vi "SwissSPAD Live_Init Settings.vi"(8 "error in (no error)":errorcluster) -> (0 "error out":errorcluster)   [LabVIEW 2021]
uses:
  SwissSPAD Live_Settings List.ctl
  SwissSPAD Live_SS2 Gate Configuration.ctl
  SwissSPAD Live_SS2 Gate Definition.ctl
  SwissSPAD Live_Gate Configuration Action.ctl
  SwissSPAD Live_SS2 DAQ Parameters 3.ctl
  SwissSPAD Live_SS3 DAQ Parameters.ctl
  SwissSPAD Live_SS3 Gate Definition.ctl
  SS3 Gate Width Definition Mode.ctl
  SwissSPAD Live_File Information.ctl
  SwissSPAD Live_FPGA Data to Display.ctl
  Phasor/Image Binning Options.ctl
  SwissSPAD Live_Image Display Options.ctl
  SwissSPAD Live_Image ROI Information.ctl
  SwissSPAD Live_SS3 Displayed Image.ctl
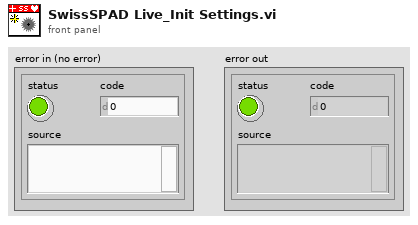
[diagram p1: front panel]
types:
  T1 = typedef "SwissSPAD Live_SS2 Gate Configuration.ctl" = cluster{"Gate Configuration":string, "Gate Offset":u32, "Gate Definition":T2}
  T2 = typedef "SwissSPAD Live_SS2 Gate Definition.ctl" = cluster{"gs_psincdec_0":u32, "gs_psincdec_1":u32, "gs_psincdec_2":u32, "gs_psincdec_3":u32, "gs_no_shift_adj_1":u32, "gs_no_shift_adj_2":u32, "gs_no_shift_adj_3":u32}
  T3 = typedef "SwissSPAD Live_Settings List.ctl" = enum16{"FPGA:Bottom Half", "FPGA:Top Half", "FPGA:Bottom Bitfile Path", "FPGA:Top Bitfile Path", "FPGA:Bottom Bitstream Version", "FPGA:Top Bitstream Version", "FPGA:Auto Reset FPGA", "FPGA:Bottom FPGA Serial Number", "FPGA:Top FPGA Serial Number", "FPGA:Detector PCB Version", "Acquisition Parameters:Microlens", "Acquisition Parameters:SS2 DAQ Parameters", "Acquisition Parameters:Gate Configuration Array", "Acquisition Parameters:SS3 DAQ Parameters", "Acquisition Parameters:Buffer Size (# 8-bit Gates)", "File Information:File Information", "File Information:# Datasets in Series", "File Information:Scrambled File Flag", "File Information:SS3 Gate Slip Correction", "File Information:SS3 Hot Pixel Mismatch Detection", "File Information:Delay between Datasets", "File Information:Save Sum of All Gates Preview", "Image Parameters:Image ROI Information", "Image Parameters:Image Binning Options", "Image Parameters:SS3 Displayed Image", "Image Parameters:Image Display Options", "Image Parameters:Use Histogram Cursors", "Image Parameter:FPGA Data to Display", "UI Settings:Histogram Bins Number", "UI Settings:Use Image Display Options", "UI Settings:Verbose Settings", "UI Settings:Verbose Saving"}
  T4 = typedef "SwissSPAD Live_Gate Configuration Action.ctl" = enum16{"Get Gate Configuration Name", "Get Configuration by Name", "Add Gate Configuration", "Delete Gate Configuration", "Rename Gate Configuration"}
  T5 = typedef "SwissSPAD Live_SS2 DAQ Parameters 3.ctl" = cluster{"10 bits":bool, "# Exposure Sequences":u32, "# 1-bit Frame per Gate":u32, "Gate Shift":u32, "# Gates per Set":u32, "# Sets":u32, "Laser Period":dbl[unit], "Sync Period":dbl[unit], "Gate Offset":u32, "Auto-adjust Gate Offset":bool, "Gate Definition":T2, "Reversed Shift":bool}
  T6 = typedef "SwissSPAD Live_SS3 DAQ Parameters.ctl" = cluster{"10 bits":bool, "# Exposure Sequences":u32, "# 1-bit Frame per Gate":u32, "Gate Shift":u32, "# Gate Pairs per Set":u32, "# Sets":u32, "Laser Period":dbl[unit], "Sync Period":dbl[unit], "Gate Offset":u32, "Auto-adjust Gate Offset":bool, "Gate Definition":T7, "Gate Width (ns)":dbl, "Reversed Shift":bool, "Intensity Mode":bool, "Gate Definition Mode":T8}
  T7 = typedef "SwissSPAD Live_SS3 Gate Definition.ctl" = cluster{"gs_psincdec_0":u32, "gs_psincdec_1":u32, "gs_no_shift_adj_1":u32, "gate_adj_2":u32}
  T8 = typedef "SS3 Gate Width Definition Mode.ctl" = enum32{"Item 0", "Item 1"}
  T9 = typedef "SwissSPAD Live_File Information.ctl" = cluster{"File Folder":path, "File Name":string, "File Index":u32, "Author":string, "Sample":string, "Compression":bool, "Compression Level":u8}
  T10 = typedef "SwissSPAD Live_FPGA Data to Display.ctl" = enum16{"Bottom FPGA", "Top FPGA", "Both"}
  T11 = typedef "Image Binning Options.ctl" = cluster{"Use Image Binning":bool, "X Bin":i32, "Y Bin":i32}
  T12 = typedef "SwissSPAD Live_Image Display Options.ctl" = cluster{"Remove Screamers":bool, "Delta":sgl, "Equalize Histogram":bool, "Percentile":sgl, "Hot Pixel Mask Image":path, "Use Hot Pixel Mask":bool}
  T13 = typedef "SwissSPAD Live_Image ROI Information.ctl" = cluster{"Save ROI Only":bool, "Left":u16, "Top":u16, "Right":u16, "Bottom":u16, "Use Current ROI":bool}
  T14 = typedef "SwissSPAD Live_SS3 Displayed Image.ctl" = enum16{"Gate 1", "Gate 2", "Gate 1 + Gate 2"}
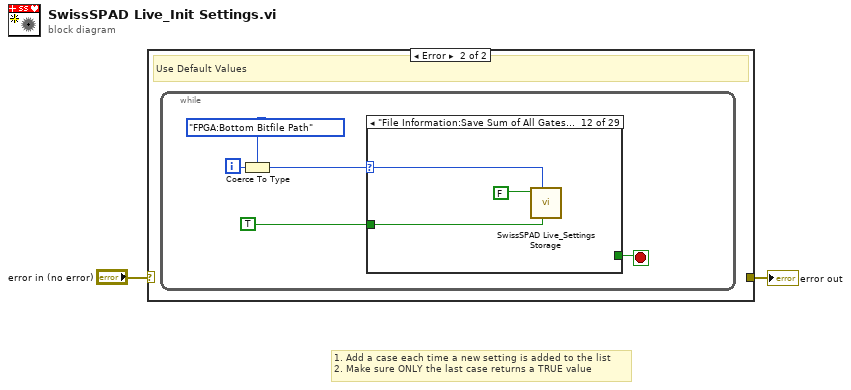
[diagram p0: block diagram]
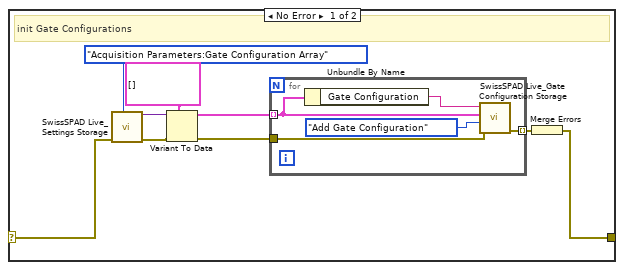
[diagram p2: hidden frame]
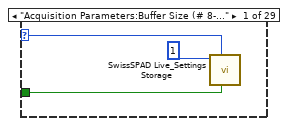
[diagram p3: hidden frame]
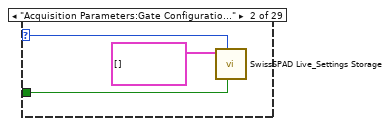
[diagram p4: hidden frame]
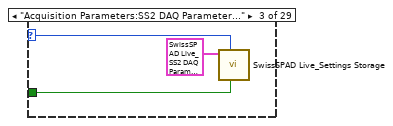
[diagram p5: hidden frame]
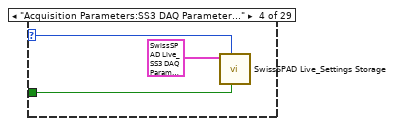
[diagram p6: hidden frame]
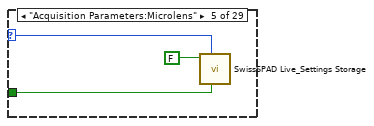
[diagram p7: hidden frame]
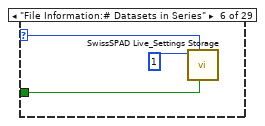
[diagram p8: hidden frame]
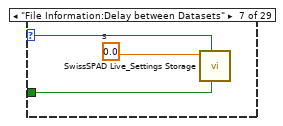
[diagram p9: hidden frame]
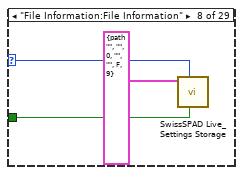
[diagram p10: hidden frame]
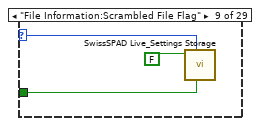
[diagram p11: hidden frame]
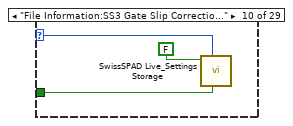
[diagram p12: hidden frame]
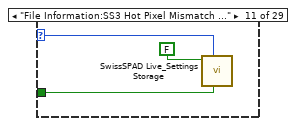
[diagram p13: hidden frame]
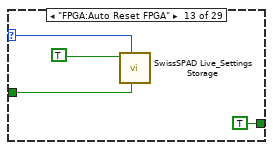
[diagram p14: hidden frame]
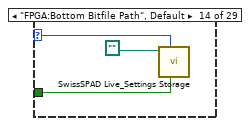
[diagram p15: hidden frame]
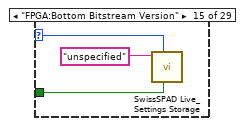
[diagram p16: hidden frame]
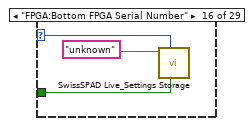
[diagram p17: hidden frame]
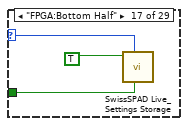
[diagram p18: hidden frame]
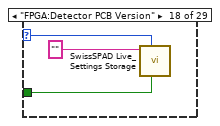
[diagram p19: hidden frame]
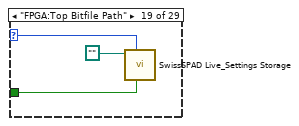
[diagram p20: hidden frame]
diagram:
  # "1. Add a case each time a new setting is added to the list\n2. Make sure ONLY the last case returns a TRUE value"
  n1 = case shown="Error" "error in (no error)" {
    selector: "error in (no error)" -> [w6 _]
    tunnel: [w5 _] -> w1
    frame No Error {
      # "init Gate Configurations"
      n2 = call "SwissSPAD Live_Settings Storage.vi"("Settings List"=SwissSPAD_Live_Settings_List."Acquisition Parameters:Gate Configuration Array", "Error In"=w6) -> ("Error Out"=w11:errorcluster, "Variant Data out"=w3:variant)  [unwired: 8 in]
      n3 = Variant To Data(error in=w11, type=T1[] [] ("Gate Configuration Definitions"), Variant=w3) -> (data=w9:T1[], error out=w8:errorcluster)
      n4 = for {
        tunnel: w9 -> [w15] mode=indexing
        tunnel: w8 -> [w13]
        tunnel: [w12] -> w7 mode=indexing
        n5 = Unbundle By Name(w15) -> ("Gate Configuration"=w16:string)
        n6 = call "SwissSPAD Live_Gate Configuration Storage.vi"("Error In"=w13, "Action"=SwissSPAD_Live_Gate_Configuration_Action."Add Gate Configuration", "Gate Configuration Definition in"=w15, "Gate Configuration Name in"=w16) -> ("Error Out"=w12:errorcluster)  [unwired: 2 in, 5 out]
      }
      n7 = Merge Errors(w7) -> (w5:errorcluster)
    }
    frame Error {
      # "Use Default Values"
      n8 = while {
        i -> [w21]
        stop <- w17 stop-if-true
        n9 = Coerce To Type(0:w21, 1:SwissSPAD_Live_Settings_List."FPGA:Bottom Bitfile Path" ("Settings List")) -> (2:w19:T3)
        n10 = case shown="\"File Information:Save Sum of All Gates Preview\"" w19 {
          selector: w19 -> [w23 w25 w29 w31 w35 w38 w41 w43 w47 w50 w53 w56 w58 w63 w66 w69 w72 w74 w78 w81 w84 w87 w90 w93 w95 w99 w102 w105 w108]
          tunnel: TRUE -> [w24 w27 w30 w33 w36 w39 w42 w45 w48 w51 w54 w57 w60 w64 w67 w70 w73 w76 w79 w82 w85 w88 w91 w94 w97 w100 w103 w106 w109]
          tunnel: [_ _ _ _ _ _ _ _ _ _ _ _ TRUE _ _ _ _ _ _ _ _ _ _ _ _ _ _ _ _] -> w17
          frame "Acquisition Parameters:Buffer Size (# 8-bit Gates)" {
            n11 = call "SwissSPAD Live_Settings Storage.vi"("Set/Get(F)"=w24, "Settings List"=w23, "Variant Data in"=u32 1 ("Buffer Size #Gates)")) -> ()  [unwired: 7 in, 2 out]
          }
          frame "Acquisition Parameters:Gate Configuration Array" {
            n12 = call "SwissSPAD Live_Settings Storage.vi"("Set/Get(F)"=w27, "Settings List"=w25, "Variant Data in"=T1[] [] ("Gate Configuration Definitions")) -> ()  [unwired: 7 in, 2 out]
          }
          frame "Acquisition Parameters:SS2 DAQ Parameters" {
            n13 = call "SwissSPAD Live_Settings Storage.vi"("Set/Get(F)"=w30, "Settings List"=w29, "Variant Data in"=T5 {"10 bits"=FALSE, "# Exposure Sequences"=100, "# 1-bit Frame per Gate"=255, "Gate Shift"=0, "# Gates per Set"=1, "# Sets"=1, "Laser Period"=0.0, "Sync Period"=0.0, "Gate Offset"=650, "Auto-adjust Gate Offset"=FALSE, "Gate Definition"={"gs_psincdec_0"=1, "gs_psincdec_1"=0, "gs_psincdec_2"=0, "gs_psincdec_3"=0, "gs_no_shift_adj_1"=65, "gs_no_shift_adj_2"=90, "gs_no_shift_adj_3"=30}, "Reversed Shift"=FALSE} ("SS2 DAQ Parameters")) -> ()  [unwired: 7 in, 2 out]
          }
          frame "Acquisition Parameters:SS3 DAQ Parameters" {
            n14 = call "SwissSPAD Live_Settings Storage.vi"("Set/Get(F)"=w33, "Settings List"=w31, "Variant Data in"=T6 {"10 bits"=FALSE, "# Exposure Sequences"=0, "# 1-bit Frame per Gate"=255, "Gate Shift"=0, "# Gate Pairs per Set"=0, "# Sets"=1, "Laser Period"=0.0, "Sync Period"=0.0, "Gate Offset"=0, "Auto-adjust Gate Offset"=FALSE, "Gate Definition"={"gs_psincdec_0"=0, "gs_psincdec_1"=0, "gs_no_shift_adj_1"=0, "gate_adj_2"=0}, "Gate Width (ns)"=0.0, "Reversed Shift"=FALSE, "Intensity Mode"=FALSE, "Gate Definition Mode"=enum."Item 0"} ("SS3 DAQ Parameters")) -> ()  [unwired: 7 in, 2 out]
          }
          frame "Acquisition Parameters:Microlens" {
            n15 = call "SwissSPAD Live_Settings Storage.vi"("Set/Get(F)"=w36, "Settings List"=w35, "Variant Data in"=FALSE) -> ()  [unwired: 7 in, 2 out]
          }
          frame "File Information:# Datasets in Series" {
            n16 = call "SwissSPAD Live_Settings Storage.vi"("Set/Get(F)"=w39, "Settings List"=w38, "Variant Data in"=1) -> ()  [unwired: 7 in, 2 out]
          }
          frame "File Information:Delay between Datasets" {
            w40 = dbl[unit] 0.0  # s
            n17 = call "SwissSPAD Live_Settings Storage.vi"("Set/Get(F)"=w42, "Settings List"=w41, "Variant Data in"=w40) -> ()  [unwired: 7 in, 2 out]
          }
          frame "File Information:File Information" {
            n18 = call "SwissSPAD Live_Settings Storage.vi"("Set/Get(F)"=w45, "Settings List"=w43, "Variant Data in"=T9 {"File Folder"=path "", "File Name"="", "File Index"=0, "Author"="", "Sample"="", "Compression"=FALSE, "Compression Level"=9} ("File Information")) -> ()  [unwired: 7 in, 2 out]
          }
          frame "File Information:Scrambled File Flag" {
            n19 = call "SwissSPAD Live_Settings Storage.vi"("Set/Get(F)"=w48, "Settings List"=w47, "Variant Data in"=FALSE) -> ()  [unwired: 7 in, 2 out]
          }
          frame "File Information:SS3 Gate Slip Correction" {
            n20 = call "SwissSPAD Live_Settings Storage.vi"("Set/Get(F)"=w51, "Settings List"=w50, "Variant Data in"=FALSE) -> ()  [unwired: 7 in, 2 out]
          }
          frame "File Information:SS3 Hot Pixel Mismatch Detection" {
            n21 = call "SwissSPAD Live_Settings Storage.vi"("Set/Get(F)"=w54, "Settings List"=w53, "Variant Data in"=FALSE) -> ()  [unwired: 7 in, 2 out]
          }
          frame "File Information:Save Sum of All Gates Preview" {
            n22 = call "SwissSPAD Live_Settings Storage.vi"("Set/Get(F)"=w57, "Settings List"=w56, "Variant Data in"=FALSE) -> ()  [unwired: 7 in, 2 out]
          }
          frame "FPGA:Auto Reset FPGA" {
            n23 = call "SwissSPAD Live_Settings Storage.vi"("Set/Get(F)"=w60, "Settings List"=w58, "Variant Data in"=TRUE) -> ()  [unwired: 7 in, 2 out]
          }
          frame "FPGA:Bottom Bitfile Path", Default {
            n24 = call "SwissSPAD Live_Settings Storage.vi"("Set/Get(F)"=w64, "Settings List"=w63, "Variant Data in"=path "") -> ()  [unwired: 7 in, 2 out]
          }
          frame "FPGA:Bottom Bitstream Version" {
            n25 = call "SwissSPAD Live_Settings Storage.vi"("Set/Get(F)"=w67, "Settings List"=w66, "Variant Data in"="unspecified") -> ()  [unwired: 7 in, 2 out]
          }
          frame "FPGA:Bottom FPGA Serial Number" {
            n26 = call "SwissSPAD Live_Settings Storage.vi"("Set/Get(F)"=w70, "Settings List"=w69, "Variant Data in"="unknown") -> ()  [unwired: 7 in, 2 out]
          }
          frame "FPGA:Bottom Half" {
            n27 = call "SwissSPAD Live_Settings Storage.vi"("Set/Get(F)"=w73, "Settings List"=w72, "Variant Data in"=TRUE) -> ()  [unwired: 7 in, 2 out]
          }
          frame "FPGA:Detector PCB Version" {
            n28 = call "SwissSPAD Live_Settings Storage.vi"("Set/Get(F)"=w76, "Settings List"=w74, "Variant Data in"="") -> ()  [unwired: 7 in, 2 out]
          }
          frame "FPGA:Top Bitfile Path" {
            n29 = call "SwissSPAD Live_Settings Storage.vi"("Set/Get(F)"=w79, "Settings List"=w78, "Variant Data in"=path "") -> ()  [unwired: 7 in, 2 out]
          }
          frame "FPGA:Top Bitstream Version" {
            n30 = call "SwissSPAD Live_Settings Storage.vi"("Set/Get(F)"=w82, "Settings List"=w81, "Variant Data in"="unspecified") -> ()  [unwired: 7 in, 2 out]
          }
          frame "FPGA:Top FPGA Serial Number" {
            n31 = call "SwissSPAD Live_Settings Storage.vi"("Set/Get(F)"=w85, "Settings List"=w84, "Variant Data in"="unknown") -> ()  [unwired: 7 in, 2 out]
          }
          frame "FPGA:Top Half" {
            n32 = call "SwissSPAD Live_Settings Storage.vi"("Set/Get(F)"=w88, "Settings List"=w87, "Variant Data in"=FALSE) -> ()  [unwired: 7 in, 2 out]
          }
          frame "Image Parameter:FPGA Data to Display" {
            n33 = call "SwissSPAD Live_Settings Storage.vi"("Set/Get(F)"=w91, "Settings List"=w90, "Variant Data in"=SwissSPAD_Live_FPGA_Data_to_Display."Bottom FPGA" ("SS3 Displayed Image 2")) -> ()  [unwired: 7 in, 2 out]
          }
          frame "Image Parameters:Image Binning Options" {
            n34 = call "SwissSPAD Live_Settings Storage.vi"("Set/Get(F)"=w94, "Settings List"=w93, "Variant Data in"=T11 {"Use Image Binning"=FALSE, "X Bin"=1, "Y Bin"=1} ("Image Binning Options")) -> ()  [unwired: 7 in, 2 out]
          }
          frame "Image Parameters:Image Display Options" {
            n35 = call "SwissSPAD Live_Settings Storage.vi"("Set/Get(F)"=w97, "Settings List"=w95, "Variant Data in"=T12 {"Remove Screamers"=FALSE, "Delta"=0.0, "Equalize Histogram"=FALSE, "Percentile"=2.0, "Hot Pixel Mask Image"=path "", "Use Hot Pixel Mask"=FALSE} ("Image Display Options")) -> ()  [unwired: 7 in, 2 out]
          }
          frame "Image Parameters:Image ROI Information" {
            n36 = call "SwissSPAD Live_Settings Storage.vi"("Set/Get(F)"=w100, "Settings List"=w99, "Variant Data in"=T13 {"Save ROI Only"=FALSE, "Left"=0, "Top"=0, "Right"=0, "Bottom"=0, "Use Current ROI"=FALSE} ("Image Information")) -> ()  [unwired: 7 in, 2 out]
          }
          frame "Image Parameters:SS3 Displayed Image" {
            n37 = call "SwissSPAD Live_Settings Storage.vi"("Set/Get(F)"=w103, "Settings List"=w102, "Variant Data in"=SwissSPAD_Live_SS3_Displayed_Image."Gate 1 + Gate 2" ("Image to Display")) -> ()  [unwired: 7 in, 2 out]
          }
          frame "Image Parameters:Use Histogram Cursors" {
            n38 = call "SwissSPAD Live_Settings Storage.vi"("Set/Get(F)"=w106, "Settings List"=w105, "Variant Data in"=TRUE) -> ()  [unwired: 7 in, 2 out]
          }
          frame "UI Settings:Histogram Bins Number" {
            n39 = call "SwissSPAD Live_Settings Storage.vi"("Set/Get(F)"=w109, "Settings List"=w108, "Variant Data in"=256) -> ()  [unwired: 7 in, 2 out]
          }
        }
      }
    }
  }
  "error out" <- w1
